vi "BooleanSchimittTrigger.vi"(8 "Lower limit":dbl, 10 "Current Value":dbl, 11 "Upper limit":dbl) -> (3 "Scmitt result":bool)   [LabVIEW 2017]
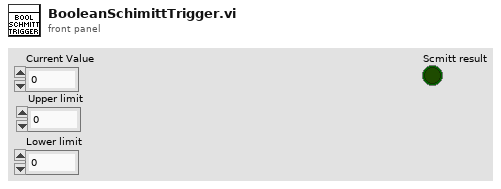
[diagram p1: front panel]
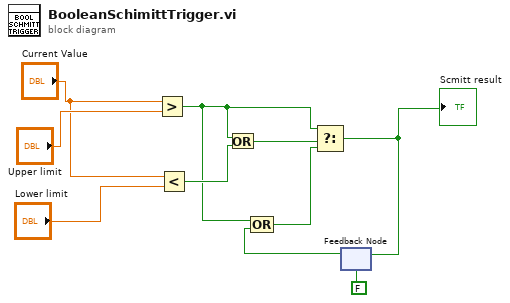
[diagram p0: block diagram]
diagram:
  n1 = Greater?(x="Current Value", y="Upper limit") -> (0:w5:bool)
  n2 = Less?(x="Current Value", y="Lower limit") -> (x < y?=w7:bool)
  n3 = Or(x=w5, y=w7) -> (x .or. y?=w6:bool)
  n4 = feedback #1(FALSE) -> (w2:bool)
  n5 = Compound Arithmetic op=OR(w5, w2) -> (w4:bool)
  n6 = Select(t=w5, s=w6, f=w4) -> (s? t:f=w3:bool)
  "Scmitt result" <- w3
  n7 = feedback-in #1(w3) -> ()
